vi "GetDBData.vi"(7 "LabVIEW Web Service Request":refnum<class "Web Request.lvclass">, 11 "TagName":string) -> (3 "Data":cluster{"TimeStamp":string, "Value":string}[](array[cluster]))   [LabVIEW 2015]
uses:
  <vilib>/wsapi/Web Request.lvclass
panel:
  # "Use the Web Service Request input terminal to call the VIs on the Web Services palette. Do not remove it from the connector pane unless you don't need access to the palette."
  # "Each additional control wired to the connector pane will be available as an input in the URL. To include an indicator in terminal-mode output (the default setting), it must also be wired to the connector pane."
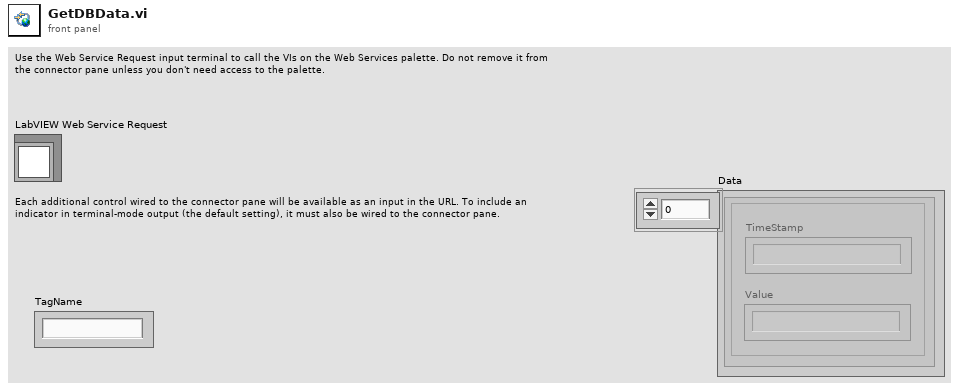
[diagram p1: front panel]
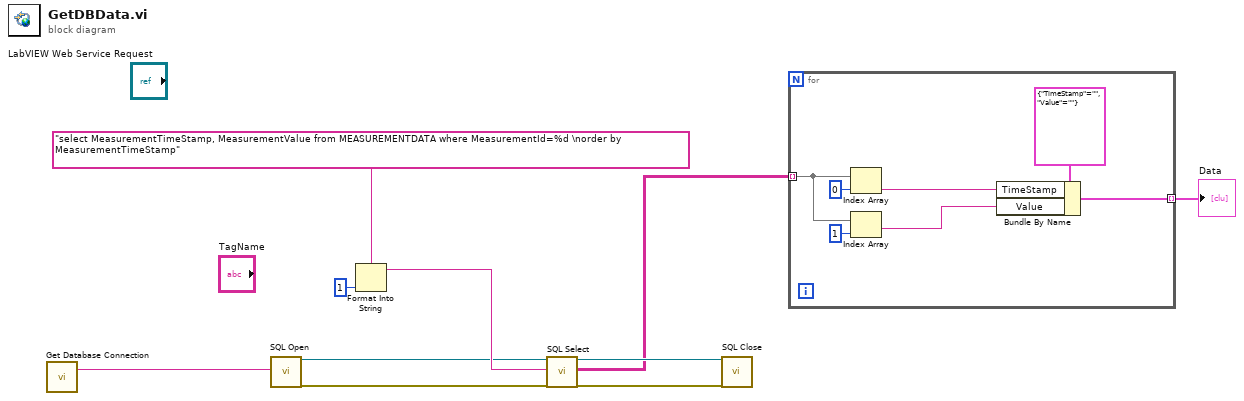
[diagram p0: block diagram]
diagram:
  n1 = call "Get Database Connection.vi"() -> ("Database  Connection String"=w4:string)  [unwired: 2 in, 1 out]
  n2 = call <vilib>:"SQL Open.vi"("ConnectionString In"=w4) -> ("Connection Out"=w8:refnum<k7>, "Error out"=w6:errorcluster)  [unwired: 17 in]
  n3 = Format Into String "Format Into String"(format string="select MeasurementTimeStamp, MeasurementValue from MEASUREMENTDATA where MeasurementId=%d \norder by MeasurementTimeStamp", 1 ("input 1")) -> (resulting string=w9:string)  [unwired: 2 in, 1 out]
  n4 = call <vilib>:"SQL Select.vi"("Connection In"=w8, "SQL Query"=w9, "Error in (no error)"=w6) -> ("Connection Out"=w7:refnum<k7>, "Data"=w2:string[][], "Error out"=w5:errorcluster)  [unwired: 14 in]
  n5 = call <vilib>:"SQL Close.vi"("Connection In"=w7, "Error in (no error)"=w5) -> ()  [unwired: 17 in, 1 out]
  n6 = for {
    tunnel: w2 -> [w15] mode=indexing
    tunnel: [w11] -> w1 mode=indexing
    n7 = Index Array(array=w15, index=0) -> (element=w14:string)
    n8 = Index Array(array=w15, index=1) -> (element=w12:string)
    n9 = Bundle By Name(cluster=cluster{"TimeStamp":string, "Value":string} {"TimeStamp"="", "Value"=""} ("Datapoint"), "TimeStamp"=w14, "Value"=w12) -> (w11:cluster{"TimeStamp":string, "Value":string})
  }
  "Data" <- w1
